vi "xboxRead.vi"() -> (0 "xboxError":errorcluster, 1 "xboxDataFull":T1)   [LabVIEW 2017]
uses:
  globalDevices.vi
  <vilib>/Utility/inputDevices.llb/joystickAcquire.vi
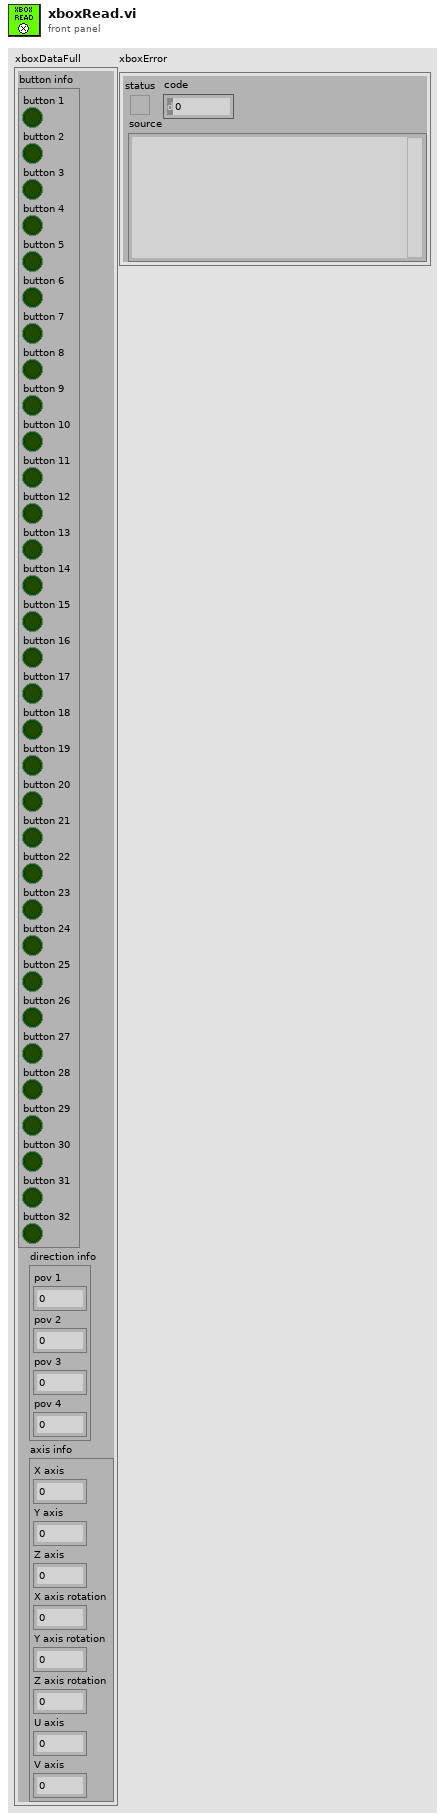
[diagram p1: front panel]
types:
  T1 = cluster{"button info":cluster{"button 1":bool, "button 2":bool, "button 3":bool, "button 4":bool, "button 5":bool, "button 6":bool, "button 7":bool, "button 8":bool, "button 9":bool, "button 10":bool, "button 11":bool, "button 12":bool, "button 13":bool, "button 14":bool, "button 15":bool, "button 16":bool, "button 17":bool, "button 18":bool, "button 19":bool, "button 20":bool, "button 21":bool, "button 22":bool, "button 23":bool, "button 24":bool, "button 25":bool, "button 26":bool, "button 27":bool, "button 28":bool, "button 29":bool, "button 30":bool, "button 31":bool, "button 32":bool}, "direction info":cluster{"pov 1":i32, "pov 2":i32, "pov 3":i32, "pov 4":i32}, "axis info":cluster{"X axis":i32, "Y axis":i32, "Z axis":i32, "X axis rotation":i32, "Y axis rotation":i32, "Z axis rotation":i32, "U axis":i32, "V axis":i32}}
  T2 = cluster{"X axis":i32, "Y axis":i32, "Z axis":i32, "X axis rotation":i32, "Y axis rotation":i32, "Z axis rotation":i32, "U axis":i32, "V axis":i32}
  T3 = cluster{"button 1":bool, "button 2":bool, "button 3":bool, "button 4":bool, "button 5":bool, "button 6":bool, "button 7":bool, "button 8":bool, "button 9":bool, "button 10":bool, "button 11":bool, "button 12":bool, "button 13":bool, "button 14":bool, "button 15":bool, "button 16":bool, "button 17":bool, "button 18":bool, "button 19":bool, "button 20":bool, "button 21":bool, "button 22":bool, "button 23":bool, "button 24":bool, "button 25":bool, "button 26":bool, "button 27":bool, "button 28":bool, "button 29":bool, "button 30":bool, "button 31":bool, "button 32":bool}
  T4 = cluster{"pov 1":i32, "pov 2":i32, "pov 3":i32, "pov 4":i32}
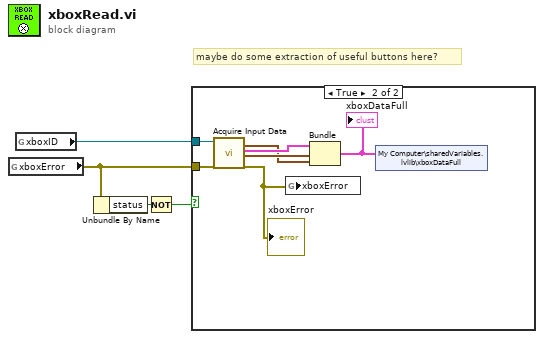
[diagram p0: block diagram]
diagram:
  # "maybe do some extraction of useful buttons here?"
  n1 = global read "globalDevices.vi" "xboxError"() -> (w3:errorcluster)
  n2 = global read "globalDevices.vi" "xboxID"() -> (w4:refnum<k1>)
  n3 = Unbundle By Name(w3) -> ("status"=w2:bool)
  n4 = Not(x=w2) -> (.not. x?=w1:bool)
  n5 = case shown="True" w1 {
    tunnel: w4 -> [_ w11]
    tunnel: w3 -> [_ w5]
    frame False {
    }
    frame True {
      n6 = call-poly <vilib>:"Acquire Input Data.vi"("device ID"=w11, "error in (no error)"=w5) -> ("axis info"=w8:T2, "button info"=w10:T3, "direction info"=w9:T4, "error out"=w6:errorcluster)  [unwired: 13 in, 1 out]
      "xboxError" <- w6
      n7 = global write "globalDevices.vi" "xboxError"(w6) -> ()
      n8 = Bundle("button info"=w10, "direction info"=w9, "axis info"=w8) -> (w7:T1)  [unwired: 1 in]
      "xboxDataFull" <- w7
      n9 = shared-variable "My Computer\\sharedVariables.lvlib\\xboxDataFull"(w7) -> ()  [unwired: 1 in, 1 out]
    }
  }
